vi "tarea ledmov.vi"() -> ()   [LabVIEW 2016]
panel:
  out "luna":bool
  in  "Cluster":cluster{"top":dbl, "left":dbl} {"left" scale=0.0..350.0; "top" scale=0.0..700.0}
  out "sol":bool
  out "tierra":bool
  in  "Stop Button":bool
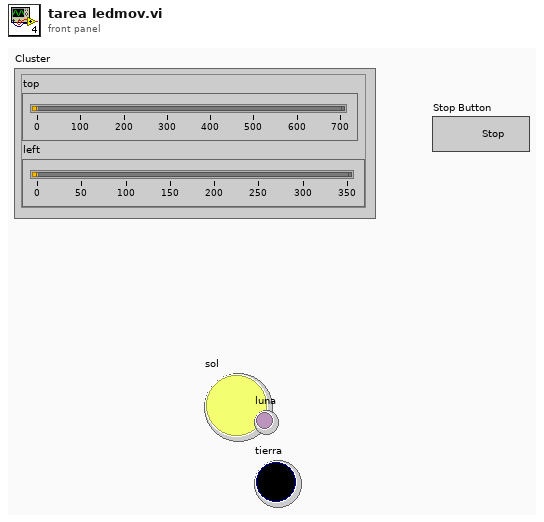
[diagram p1: front panel]
types:
  T1 = typedef "LVPositionTypeDef.ctl" = cluster{"Left":i32, "Top":i32}
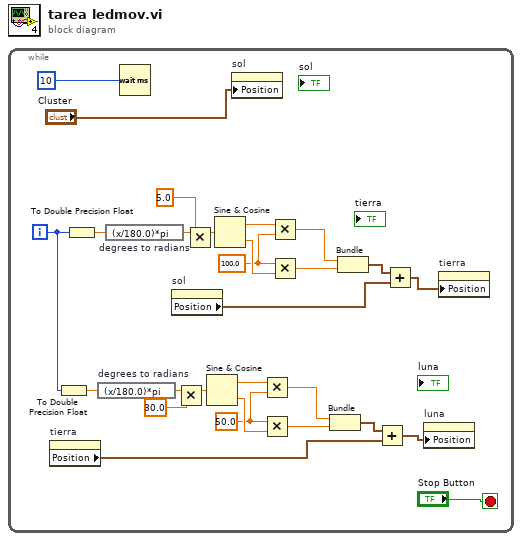
[diagram p0: block diagram]
diagram:
  n1 = while {
    i -> [w5]
    stop <- "Stop Button" stop-if-true
    w12 = 50.0 ("y")
    w23 = 100.0 ("y")
    n2 = property on="tierra" class="Bool (strict)"() -> ("Position"=w7:T1)  [unwired: 2 in, 2 out]
    n3 = To Double Precision Float(number=w5) -> (double precision float=w8:dbl)
    n4 = To Double Precision Float(number=w5) -> (double precision float=w18:dbl)
    n5 = expression code="(x/180.0)*pi" "degrees to radians"(w8) -> (w15:dbl)
    n6 = expression code="(x/180.0)*pi" "degrees to radians"(w18) -> (w26:dbl)
    n7 = Wait (ms)(milliseconds to wait=u32 10) -> ()  [unwired: 1 out]
    n8 = property on="sol" class="Bool (strict)"() -> ("Position"=w16:T1)  [unwired: 2 in, 2 out]
    n9 = Multiply(x=w15, y=30.0) -> (x*y=w4:dbl)
    n10 = Multiply(x=w26, y=5.0) -> (x*y=w2:dbl)
    n11 = Sine & Cosine(0:w4) -> (1:w14:dbl, 2:w13:dbl)
    n12 = Sine & Cosine(0:w2) -> (1:w25:dbl, 2:w24:dbl)
    n13 = property on="sol" class="Bool (strict)"("Position"="Cluster") -> ()  [unwired: 2 in, 2 out]
    n14 = Multiply(x=w14, y=w12) -> (x*y=w11:dbl)
    n15 = Multiply(x=w12, y=w13) -> (x*y=w10:dbl)
    n16 = Multiply(x=w25, y=w23) -> (x*y=w22:dbl)
    n17 = Multiply(x=w23, y=w24) -> (x*y=w21:dbl)
    n18 = Bundle(w11, w10) -> (w9:cluster{dbl, dbl})  [unwired: 1 in]
    n19 = Bundle(w22, w21) -> (w20:cluster{dbl, dbl})  [unwired: 1 in]
    n20 = Add(x=w9, y=w7) -> (x+y=w6:cluster{dbl, dbl})
    n21 = Add(x=w20, y=w16) -> (x+y=w19:cluster{dbl, dbl})
    n22 = property on="luna" class="Bool (strict)"("Position"=w6) -> ()  [unwired: 2 in, 2 out]
    n23 = property on="tierra" class="Bool (strict)"("Position"=w19) -> ()  [unwired: 2 in, 2 out]
  }
